vi "PhotonPipelineResult_GetBestTargetById.vi"(9 "PhotonPipelineResult_REF":T7, 11 "FiducialId":i32) -> (1 "Target Found":bool, 3 "PhotonTrackedTarget":T1={"Yaw"=0.0, "Pitch"=0.0, "Area"=0.0, "Skew"=0.0, "MinAreaRectCorners"=[], "BestCameraToTarget"={"TRANSLATION3D"={"X"=0.0, "Y"=0.0, "Z"=0.0}, "ROTATION3D"={"Q_quaternion"={"R"=1.0, "V"=[0.0, 0.0, 0.0]}}, "XF"=FALSE}, "FiiducialId"=0, "AltCameraToTarget"={"TRANSLATION3D"={"X"=0.0, "Y"=0.0, "Z"=0.0}, "ROTATION3D"={"Q_quaternion"={"R"=0.0, "V"=[0.0, 0.0, 0.0]}}, "XF"=FALSE}, "PoseAmbiguity"=0.0, "DetectedCorners"=[]} {"AltCameraToTarget"."TRANSLATION3D"."Z" format="%14.3f"; "AltCameraToTarget"."TRANSLATION3D"."Y" format="%14.3f"; "AltCameraToTarget"."TRANSLATION3D"."X" format="%14.3f"; "BestCameraToTarget"."TRANSLATION3D"."Z" format="%14.3f"; "BestCameraToTarget"."TRANSLATION3D"."Y" format="%14.3f"; "BestCameraToTarget"."TRANSLATION3D"."X" format="%14.3f"}, 4 "Target Index":i32)   [LabVIEW 2019, in "PhotonVisionLib.lvlib"]
doc: "Returns the best target in this pipeline result filtered by fiducial ID (April tag numer). If there are no targets, or no targets with this fiducial ID, this method will return an empty target. IF more than 1 targets have the same fiducial ID, the best target is determined by the sort mode in the PhotonVision UI.\n\nInputs:\n - PipelineResult -- Parsed PipelineResult cluster.\n - Fiducial ID -- The April tag number being searched for.\n\nOutputs:\n - TrackedTarget -- Cluster containing the best target\n - TargetFound -- TRUE if a target matching the search criteria exits.\n - TargetIndex -- Index into the targets array of the best target matching the search criteria."
uses:
  PhotonVisionLib.lvlib
  TypeDef/PhotonPipelineResultType.ctl
  TypeDef/PhotonTrackedTargetType.ctl
  TypeDef/TargetCornerType.ctl
  <vilib>/Rock Robotics/WPI/ThirdParty/JAS_Junk/TrajLib/TypeDef/TRANSFORM3D.ctl
  <vilib>/Rock Robotics/WPI/ThirdParty/JAS_Junk/TrajLib/TypeDef/TRANSLATION3D.ctl
  <vilib>/Rock Robotics/WPI/ThirdParty/JAS_Junk/TrajLib/TypeDef/ROTATION3D.ctl
  <vilib>/Rock Robotics/WPI/ThirdParty/JAS_Junk/TrajLib/TypeDef/QUATERNION.ctl
  TypeDef/PhotonMultiTargetPNPResultType.ctl
  TypeDef/PhotonPNPResultType.ctl
  <vilib>/Rock Robotics/WPI/ThirdParty/JAS_Junk/TrajLib/Trajectory_Library.lvlib
  Ref/PhotonPipelineResult_REF.ctl
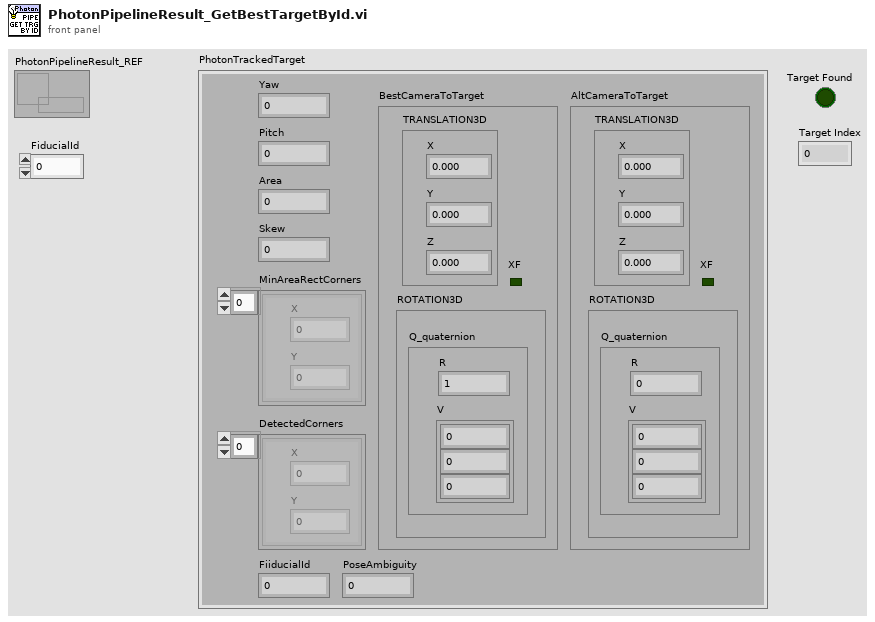
[diagram p1: front panel]
types:
  T1 = typedef "PhotonVisionLib.lvlib/PhotonTrackedTargetType.ctl" = cluster{"Yaw":dbl, "Pitch":dbl, "Area":dbl, "Skew":dbl, "MinAreaRectCorners":T2[], "BestCameraToTarget":T3, "FiiducialId":i32, "AltCameraToTarget":T3, "PoseAmbiguity":dbl, "DetectedCorners":T2[]}
  T2 = typedef "PhotonVisionLib.lvlib/TargetCornerType.ctl" = cluster{"X":dbl, "Y":dbl}
  T3 = typedef "Trajectory_Library.lvlib/TRANSFORM3D.ctl" = cluster{"TRANSLATION3D":T4, "ROTATION3D":T5, "XF":bool}
  T4 = typedef "Trajectory_Library.lvlib/TRANSLATION3D.ctl" = cluster{"X":dbl, "Y":dbl, "Z":dbl}
  T5 = typedef "Trajectory_Library.lvlib/ROTATION3D.ctl" = cluster{"Q_quaternion":T6}
  T6 = typedef "Trajectory_Library.lvlib/QUATERNION.ctl" = cluster{"R":dbl, "V":dbl[]}
  T7 = typedef "PhotonVisionLib.lvlib/PhotonPipelineResult_REF.ctl" = refnum<data-value>
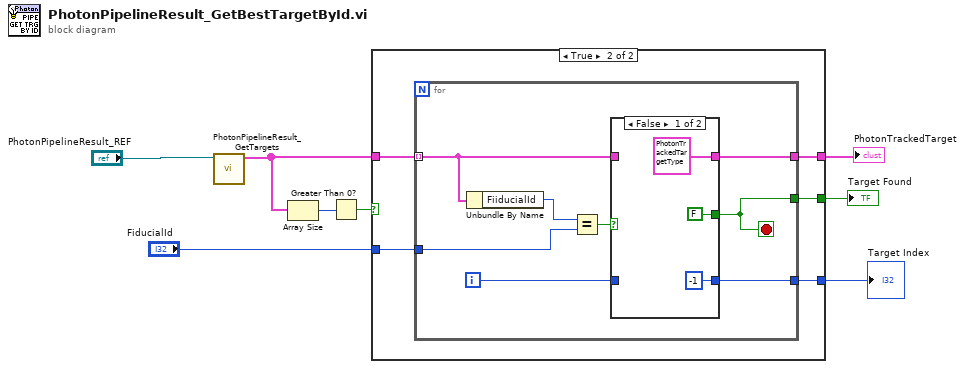
[diagram p0: block diagram]
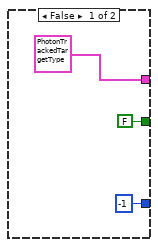
[diagram p2: hidden frame]
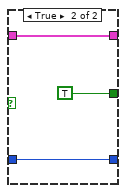
[diagram p3: hidden frame]
diagram:
  n1 = call "PhotonPipelineResult_GetTargets.vi"("PhotonPipelineResult_REF"="PhotonPipelineResult_REF") -> ("Targets"=w1:T1[])  [unwired: 10 in]
  n2 = Array Size(array=w1) -> (size(s)=w4:i32)
  n3 = Greater Than 0?(x=w4) -> (x > 0?=w3:bool)
  n4 = case shown="True" w3 {
    tunnel: "FiducialId" -> [_ w16]
    tunnel: [FALSE w15] -> w7
    tunnel: [T1 {"Yaw"=0.0, "Pitch"=0.0, "Area"=0.0, "Skew"=0.0, "MinAreaRectCorners"=[], "BestCameraToTarget"={"TRANSLATION3D"={"X"=0.0, "Y"=0.0, "Z"=0.0}, "ROTATION3D"={"Q_quaternion"={"R"=1.0, "V"=[0.0, 0.0, 0.0]}}, "XF"=FALSE}, "FiiducialId"=0, "AltCameraToTarget"={"TRANSLATION3D"={"X"=0.0, "Y"=0.0, "Z"=0.0}, "ROTATION3D"={"Q_quaternion"={"R"=1.0, "V"=[0.0, 0.0, 0.0]}}, "XF"=FALSE}, "PoseAmbiguity"=0.0, "DetectedCorners"=[]} ("PhotonTrackedTarget") w14] -> w6
    tunnel: w1 -> [_ w13]
    tunnel: [-1 w12] -> w5
    frame False {
    }
    frame True {
      n5 = for {
        tunnel: w16 -> [w24]
        tunnel: w13 -> [w20] mode=indexing
        tunnel: [w18] -> w14
        tunnel: [w19] -> w15
        tunnel: [w17] -> w12
        i -> [w22]
        stop <- w19 stop-if-true
        n6 = Unbundle By Name(w20) -> ("FiiducialId"=w21:i32)
        n7 = Equal?(x=w21, y=w24) -> (x = y?=w23:bool)
        n8 = case shown="False" w23 {
          tunnel: w22 -> [_ w28]
          tunnel: w20 -> [_ w29]
          tunnel: [FALSE TRUE] -> w19
          tunnel: [T1 {"Yaw"=0.0, "Pitch"=0.0, "Area"=0.0, "Skew"=0.0, "MinAreaRectCorners"=[], "BestCameraToTarget"={"TRANSLATION3D"={"X"=0.0, "Y"=0.0, "Z"=0.0}, "ROTATION3D"={"Q_quaternion"={"R"=1.0, "V"=[0.0, 0.0, 0.0]}}, "XF"=FALSE}, "FiiducialId"=0, "AltCameraToTarget"={"TRANSLATION3D"={"X"=0.0, "Y"=0.0, "Z"=0.0}, "ROTATION3D"={"Q_quaternion"={"R"=1.0, "V"=[0.0, 0.0, 0.0]}}, "XF"=FALSE}, "PoseAmbiguity"=0.0, "DetectedCorners"=[]} ("PhotonTrackedTarget") w29] -> w18
          tunnel: [-1 w28] -> w17
          frame False {
          }
          frame True {
          }
        }
      }
    }
  }
  "PhotonTrackedTarget" <- w6
  "Target Found" <- w7
  "Target Index" <- w5
